vi "Get Display Text.vi"(8 "error in (no error)":errorcluster, 11 "Data Item in":refnum<class "Data Item.lvclass">) -> (0 "error out":errorcluster, 1 "Detail Text":string, 2 "Display Name":string, 3 "Data Item out":refnum<class "Data Item.lvclass">)   [LabVIEW 2026, in "VILab.lvlib" / "Data Item.lvclass"]
uses:
  Data Item.lvclass
  Data Item.lvclass/Data Item.ctl
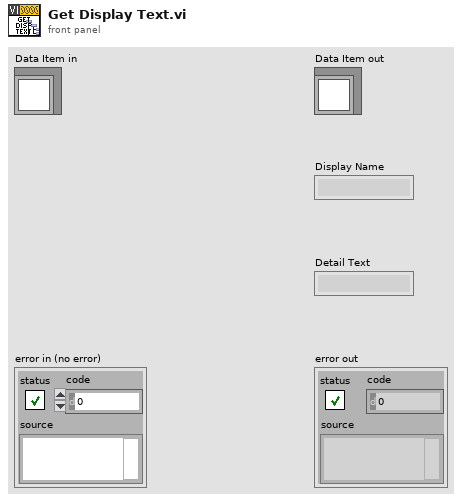
[diagram p1: front panel]
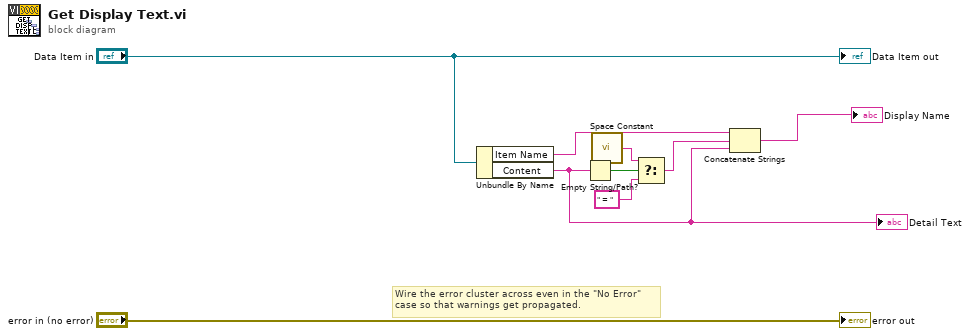
[diagram p0: block diagram]
diagram:
  # "Wire the error cluster across even in the \"No Error\"\ncase so that warnings get propagated."
  n1 = Unbundle By Name("Data Item in") -> ("Item Name"=w1:string, "Content"=w6:string)
  "Detail Text" <- w6
  n2 = Empty String/Path?(string/path=w6) -> (empty?=w5:bool)
  n3 = call <vilib>:"Space Constant.vi"() -> ("String"=w4:string)
  n4 = Select(t=w4, s=w5, f=" = ") -> (s? t:f=w2:string)
  n5 = Concatenate Strings(w1, w2, w6) -> (→"Display Name":string)
  "error out" <- "error in (no error)"
  "Data Item out" <- "Data Item in"
